vi "AlliGator Get Phasor Plot Calibration Message String.vi"(5 "Calibration CPU (s)":dbl, 6 "Calibration Phasor":T21, 7 "Message in":string, 8 "error in (no error)":errorcluster, 9 "AlliGator Phasor Calibration Options":T2={"Phasor Frequency"=0.0, "Phasor Calibration"={"Calibration Lifetime"=1e-09, "Calibration Type"=enum."Single Phasor", "Calibration Map Algorithm"=enum."Simple Search", "Use Backup Calibration if needed"=TRUE, "Backup Calibration Type"=enum."Single Calibration"}}, 10 "Phasor Calibration Map Characteristics":T1={"Phasor Frequency"=80000000.0, "Calibration Lifetime"=1e-09, "Map Resolution X"=0, "Map Resolution Y"=0, "Empty Map"=FALSE}, 11 "Phasor Plot Parameters":T5={"Phasor Frequency"=0.0, "Decay Preprocessing Options & Parameters"={"Background Subtraction Parameters"={"Background Definition Range"={"Min Gate"=0.0, "Max Gate"=0.0}, "Baseline Subtraction Method"=enum."Mean", "Background Subtraction?"=FALSE, "Background File"=path "", "Background Constant"=0.0, "Background Scaling Factor"=1.0, "Background Pile-up Correction"=FALSE, "Background Pixel Well Capacity"=1}, "Decay Preprocessing Parameters"={"Background Subtraction"=FALSE, "Straighten Decay"=FALSE, "Reverse Gates"=FALSE, "1-Normalized Decay"=FALSE, "Smoothen Decay"=FALSE, "Smoothing Parameter"=0.0, "Shift Decay"=FALSE, "Decay Shift Parameters"={"Type"=enum."Default", "Shift"=0.0, "Threshold"=0.0, "Rotate"=FALSE}, "Extrapolate Decay"=FALSE, "Additional Points"=0, "Head Fraction"=0.0, "Pixel-Normalize Decay"=FALSE, "Use Periodicity"=FALSE, "Use Cursors"=FALSE, "Tail Fraction"=0.0, "Use Decay Pre-Processing"=TRUE, "Fold Decay"=FALSE, "# Folds"=1, "[0-1]-Normalized Decay"=FALSE}, "Preprocessing Steps Order"=[]}, "FLI Dataset Modified"=FALSE, "Source Image Settings"={"Low Count Pixels Rejection Options"={"Background Low Threshold Factor"=0.0, "Fixed Low Background Threshold"=0.0, "Reject Low Count Pixels"=FALSE, "Low Percentile"=0.0}, "High Count Pixels Rejection Options"={"Background High Threshold Factor"=0.0, "Fixed High Background Threshold"=0.0, "Reject High Count Pixels"=FALSE, "High Percentile"=0.0}}, "Data Information"={"Gate Width"=0.0, "Gate Separation"=0.0, "Step (Gate Separation)"=0, "Laser Period"=0.0, "SYNC Period"=0.0, "Channel Name"=0, "Channel Arithmetic"=enum."None", "Pile-up Correction"=FALSE, "Pixel Well Capacity"=1, "Dataset Scaling Factor"=1.0}, "Phasor Plot"={"Phasor Plot Smoothing Options"={"Use Phasor Plot Smoothing"=FALSE, "Kernel Type"=enum."Uniform", "Bin"=1, "Algorithm"=enum."Rapid"}, "Phasor Plot Size"={"H"=0, "V"=0, "Margin"=0.0}, "Selected Image ROI(s)"=FALSE, "All Image ROIs"=FALSE, "Selected Source Image ROI"=0, "Source Image ROIs"=[]}} {"Phasor Plot"."Source Image ROIs"."ROI Descriptor"."Contours"."Type" items=["No Selection", "Point", "Line", "Rectangle", "Oval", "Polygon", "Freehand Region", "Annulus", "Unused2", "Unused3", "Broken Line", "Freehand Line", "Rotated Rectangle"]; "Phasor Plot"."Phasor Plot Smoothing Options"."Bin" min=1 step=2; "Data Information"."Dataset Scaling Factor" min=0.0; "Data Information"."Pixel Well Capacity" min=1 step=1; "Data Information"."Channel Name" items=["Gate"]; "Source Image Settings"."High Count Pixels Rejection Options"."High Percentile" min=0.0 max=100.0; "Source Image Settings"."Low Count Pixels Rejection Options"."Low Percentile" min=0.0 max=100.0; "Decay Preprocessing Options & Parameters"."Decay Preprocessing Parameters"."# Folds" min=1; "Decay Preprocessing Options & Parameters"."Background Subtraction Parameters"."Background Pixel Well Capacity" min=1 step=1; "Phasor Frequency" min=-2147483648.0 max=2147483647.0}) -> (0 "error out":errorcluster, 3 "Message out":string)   [LabVIEW 2021, in "AlliGator Phasor Plot.lvlib"]
doc: "Builds string specifying which phasor calibration is used."
uses:
  AlliGator Phasor Plot.lvlib
  Phasor/Calibration Phasor (m, phi).ctl
  AlliGator Phasor Plot Parameters v2.ctl
  Decay Analysis/Decay Preprocessing/AlliGator Decay Preprocessing Options.ctl
  Decay Analysis/Decay Preprocessing/AlliGator Background Subtraction Parameters.ctl
  Decay Analysis/Decay Preprocessing/AlliGator Baseline Subtraction Method.ctl
  Decay Analysis/Decay Preprocessing/AlliGator Decay Preprocessing Parameters.ctl
  Graphs/XY Graph/XY Graph Plot Shift Parameters.ctl
  Graphs/XY Graph/XY Graph Plot Shift Method.ctl
  Settings/AlliGator Low Count Pixels Rejection Options.ctl
  Settings/AlliGator High Count Pixels Rejection Options.ctl
  Settings/AlliGator Gate Arithmetic.ctl
  AlliGator Phasor Plot Smoothing Options.ctl
  Arrays/Kernel Type.ctl
  Arrays/Smoothing Algorithm.ctl
  AlliGator Phasor Plot Size.ctl
  Image/Named ROI Description.ctl
  Phasor Calibration/AlliGator Phasor Calibration Options.ctl
  Phasor/Phasor Calibration Type.ctl
  Phasor Calibration/AlliGator Calibration Map Algorithm.ctl
  Phasor/Phasor Calibration Map Characteristics.ctl
  AlliGator Abridged Phasor Plot Parameters v2.ctl
  Arrays/Arrays.lvlib
  Phasor/Phasor.lvlib
  Phasor Calibration/AlliGator Phasor Calibration.lvlib
  Variant/Variant.lvlib
  Decay Analysis/Decay Preprocessing/AlliGator Decay Preprocessing.lvlib
  Graphs/XY Graph/XY Graph Add-Ons.lvlib
  Settings/AlliGator Settings.lvlib
  Image/Image.lvlib
panel:
  # "see the AlliGator License on the block diagram (Ctrl+E or Window:Show Block Diagram)"
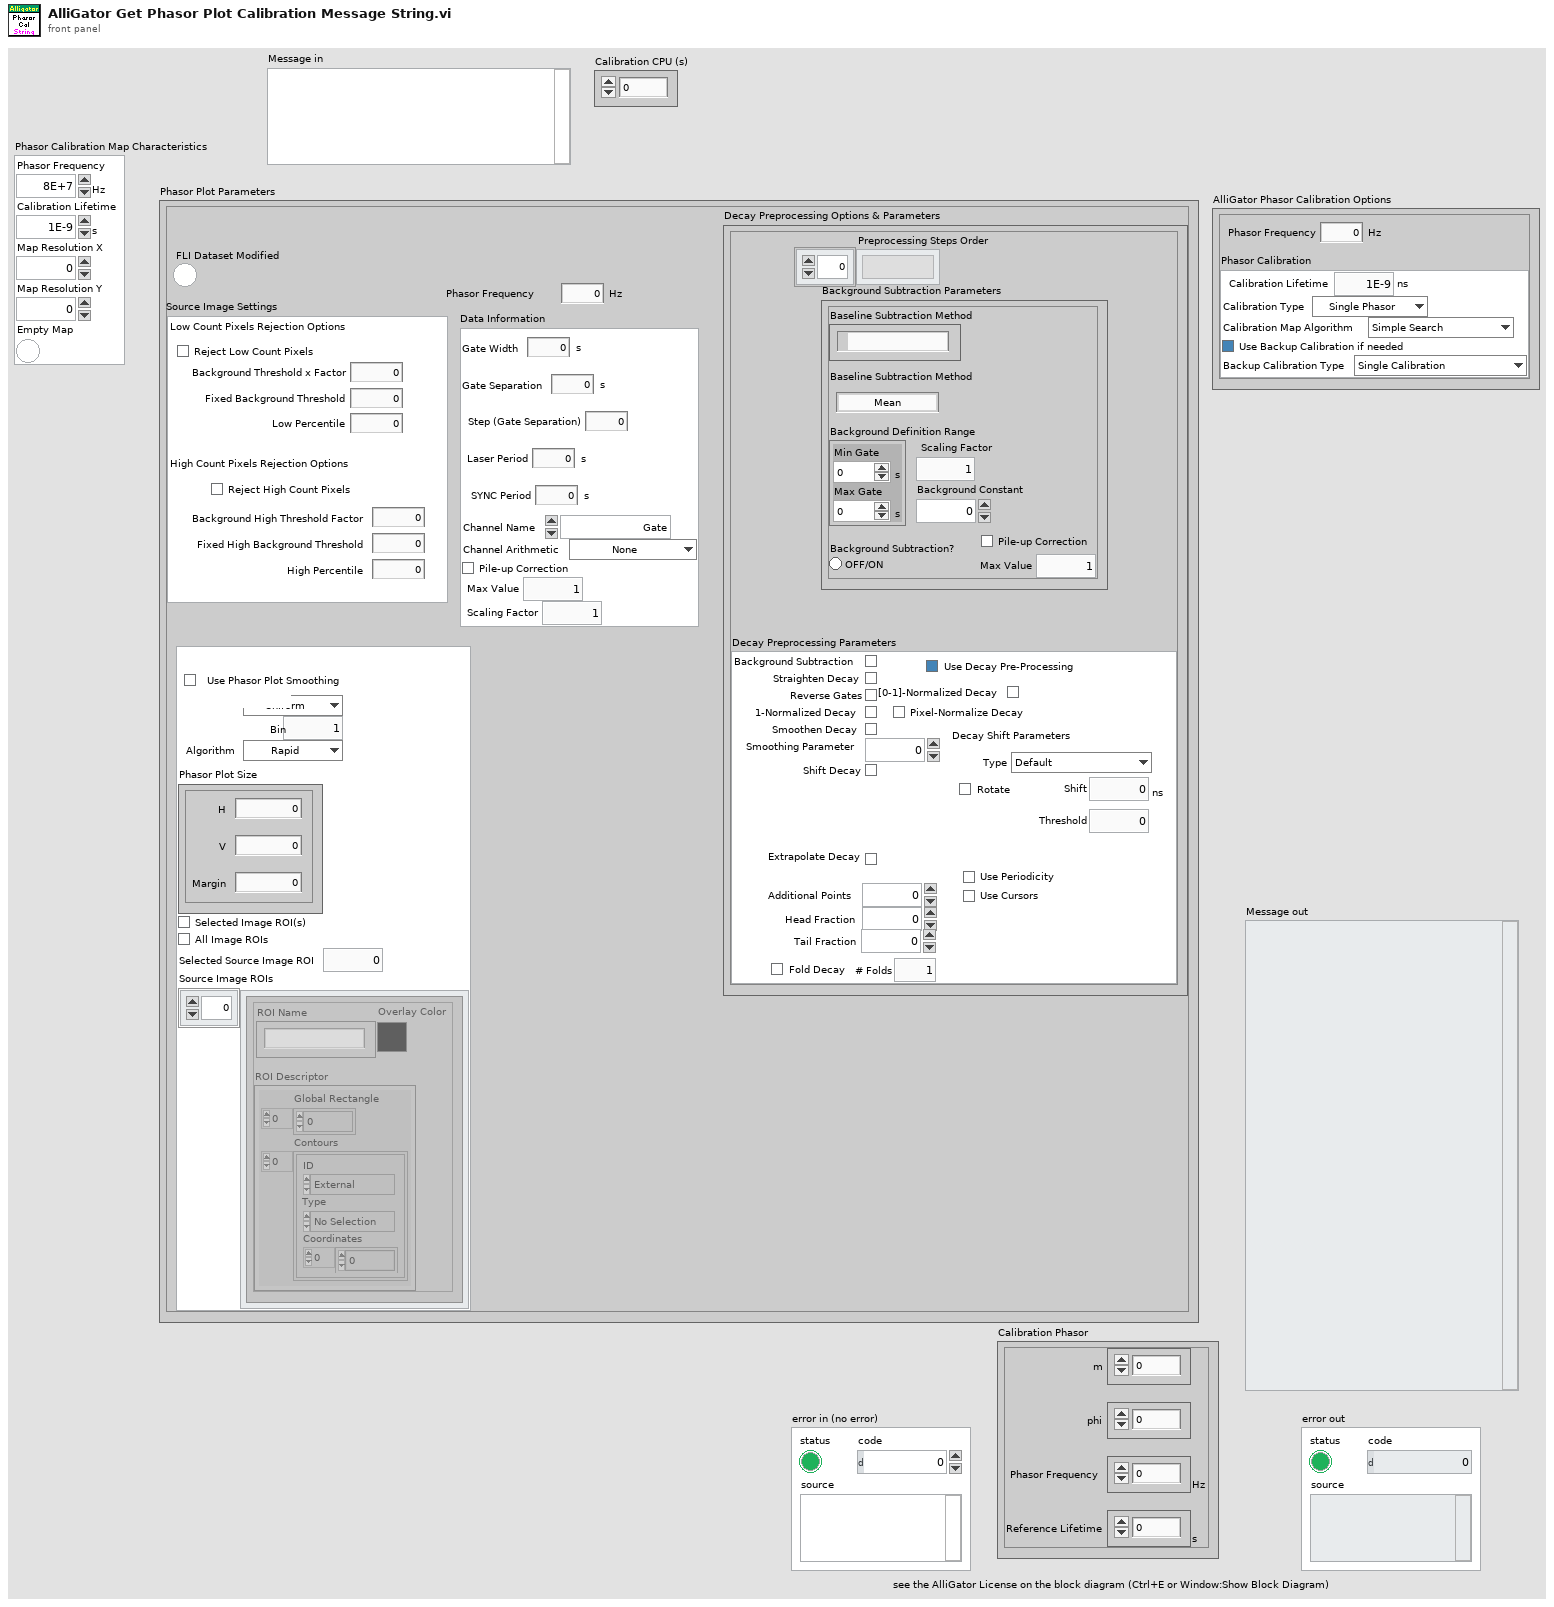
[diagram p1: front panel]
types:
  T1 = typedef "Phasor.lvlib/Phasor Calibration Map Characteristics.ctl" = cluster{"Phasor Frequency":dbl[unit], "Calibration Lifetime":dbl[unit], "Map Resolution X":i32, "Map Resolution Y":i32, "Empty Map":bool}
  T2 = typedef "AlliGator Phasor Calibration.lvlib/AlliGator Phasor Calibration Options.ctl" = cluster{"Phasor Frequency":dbl[unit], "Phasor Calibration":cluster{"Calibration Lifetime":dbl[unit], "Calibration Type":T3, "Calibration Map Algorithm":T4, "Use Backup Calibration if needed":bool, "Backup Calibration Type":enum16{"Single Calibration", "Nearest Valid Calibration"}}}
  T3 = typedef "Phasor.lvlib/Phasor Calibration Type.ctl" = enum16{"None", "Single Phasor", "Phasor Series", "Phasor Map"}
  T4 = typedef "AlliGator Phasor Calibration.lvlib/AlliGator Calibration Map Algorithm.ctl" = enum16{"Simple Search", "Min Distance"}
  T5 = typedef "AlliGator Phasor Plot.lvlib/AlliGator Phasor Plot Parameters v2.ctl" = cluster{"Phasor Frequency":dbl[unit], "Decay Preprocessing Options & Parameters":T6, "FLI Dataset Modified":bool, "Source Image Settings":cluster{"Low Count Pixels Rejection Options":T12, "High Count Pixels Rejection Options":T13}, "Data Information":cluster{"Gate Width":dbl[unit], "Gate Separation":dbl[unit], "Step (Gate Separation)":i32, "Laser Period":dbl[unit], "SYNC Period":dbl[unit], "Channel Name":u16, "Channel Arithmetic":T14, "Pile-up Correction":bool, "Pixel Well Capacity":u32, "Dataset Scaling Factor":dbl}, "Phasor Plot":cluster{"Phasor Plot Smoothing Options":T15, "Phasor Plot Size":T18, "Selected Image ROI(s)":bool, "All Image ROIs":bool, "Selected Source Image ROI":i32, "Source Image ROIs":T19[]}}
  T6 = typedef "AlliGator Decay Preprocessing.lvlib/AlliGator Decay Preprocessing Options.ctl" = cluster{"Background Subtraction Parameters":T7, "Decay Preprocessing Parameters":T9, "Preprocessing Steps Order":string[]}
  T7 = typedef "AlliGator Decay Preprocessing.lvlib/AlliGator Background Subtraction Parameters.ctl" = cluster{"Background Definition Range":cluster{"Min Gate":dbl[unit], "Max Gate":dbl[unit]}, "Baseline Subtraction Method":T8, "Background Subtraction?":bool, "Background File":path, "Background Constant":dbl, "Background Scaling Factor":dbl, "Background Pile-up Correction":bool, "Background Pixel Well Capacity":u32}
  T8 = typedef "AlliGator Decay Preprocessing.lvlib/AlliGator Baseline Subtraction Method.ctl" = enum16{"Mean", "Min", "Square Gated Single-Exponential", "File", "Constant"}
  T9 = typedef "AlliGator Decay Preprocessing.lvlib/AlliGator Decay Preprocessing Parameters.ctl" = cluster{"Background Subtraction":bool, "Straighten Decay":bool, "Reverse Gates":bool, "1-Normalized Decay":bool, "Smoothen Decay":bool, "Smoothing Parameter":dbl, "Shift Decay":bool, "Decay Shift Parameters":T10, "Extrapolate Decay":bool, "Additional Points":u32, "Head Fraction":dbl, "Pixel-Normalize Decay":bool, "Use Periodicity":bool, "Use Cursors":bool, "Tail Fraction":dbl, "Use Decay Pre-Processing":bool, "Fold Decay":bool, "# Folds":u32, "[0-1]-Normalized Decay":bool}
  T10 = typedef "XY Graph Add-Ons.lvlib/XY Graph Plot Shift Parameters.ctl" = cluster{"Type":T11, "Shift":dbl[unit], "Threshold":dbl, "Rotate":bool}
  T11 = typedef "XY Graph Add-Ons.lvlib/XY Graph Plot Shift Method.ctl" = enum16{"Default", "CFD", "Threshold", "Cross-Correlation"}
  T12 = typedef "AlliGator Settings.lvlib/AlliGator Low Count Pixels Rejection Options.ctl" = cluster{"Background Low Threshold Factor":dbl, "Fixed Low Background Threshold":dbl, "Reject Low Count Pixels":bool, "Low Percentile":dbl}
  T13 = typedef "AlliGator Settings.lvlib/AlliGator High Count Pixels Rejection Options.ctl" = cluster{"Background High Threshold Factor":dbl, "Fixed High Background Threshold":dbl, "Reject High Count Pixels":bool, "High Percentile":dbl}
  T14 = typedef "AlliGator Settings.lvlib/AlliGator Gate Arithmetic.ctl" = enum16{"None", "INT-G2", "G2/INT*<INT>", "(1 - G2/INT)*<INT>"}
  T15 = typedef "AlliGator Phasor Plot.lvlib/AlliGator Phasor Plot Smoothing Options.ctl" = cluster{"Use Phasor Plot Smoothing":bool, "Kernel Type":T16, "Bin":i32, "Algorithm":T17}
  T16 = typedef "Arrays.lvlib/Kernel Type.ctl" = enum16{"Uniform", "Bilinear", "Gaussian"}
  T17 = typedef "Arrays.lvlib/Smoothing Algorithm.ctl" = enum16{"Rapid", "Thorough"}
  T18 = typedef "AlliGator Phasor Plot.lvlib/AlliGator Phasor Plot Size.ctl" = cluster{"H":i32, "V":i32, "Margin":dbl}
  T19 = typedef "Image.lvlib/Named ROI Description.ctl" = cluster{"ROI Descriptor":T20, "ROI Name":string, "Overlay Color":u32}
  T20 = typedef "ROI Descriptor" = cluster{"Global Rectangle":i32[], "Contours":cluster{"ID":enum32{"External", "Internal"}, "Type":u32, "Coordinates":i32[]}[]}
  T21 = typedef "Phasor.lvlib/Calibration Phasor (m, phi).ctl" = cluster{"m":dbl, "phi":dbl, "Phasor Frequency":dbl[unit], "Reference Lifetime":dbl[unit]}
  T22 = typedef "AlliGator Phasor Plot.lvlib/AlliGator Abridged Phasor Plot Parameters v2.ctl" = cluster{"Phasor Frequency":dbl[unit], "Use Gate Center":bool, "Phasor Plot Smoothing Options":T15, "Selected Image ROI(s)":bool, "All Image ROIs":bool, "Calibration Lifetime":dbl[unit], "Calibration Type":T3, "Phasor Plot Size":T18, "Calibration Map Algorithm":T4, "Use Backup Calibration if needed":bool, "Backup Calibration Type":enum16{"Single Calibration", "Nearest Valid Calibration"}}
  T23 = enum16{"Single Calibration", "Nearest Valid Calibration"}
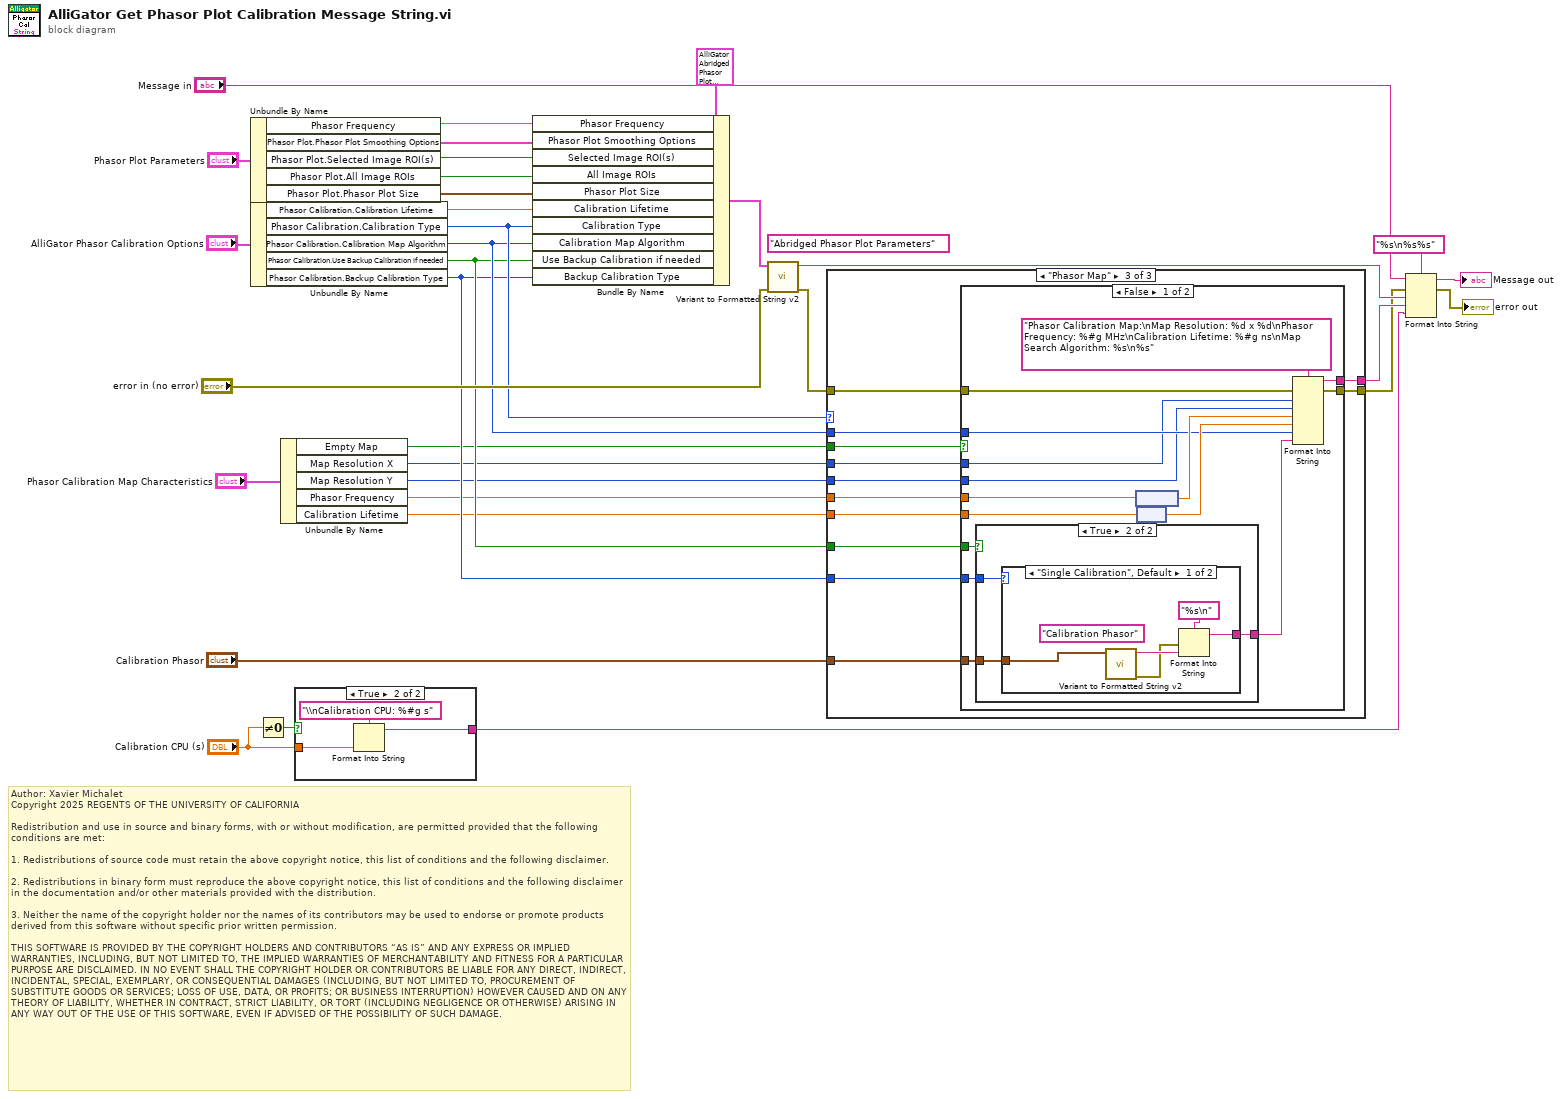
[diagram p0: block diagram]
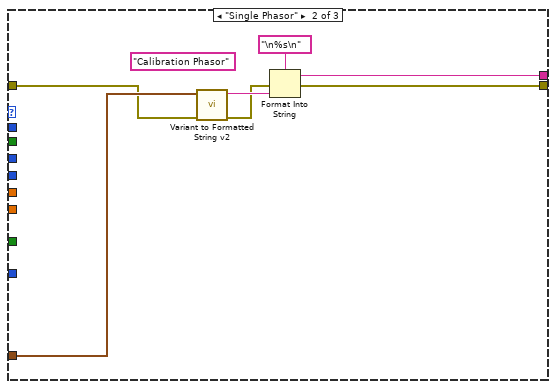
[diagram p4: hidden frame]
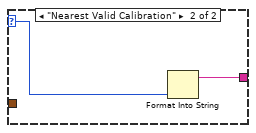
[diagram p6: hidden frame]
diagram:
  (unwired) "Abridged Phasor Plot Parameters" ("Label")
  # "Author: Xavier Michalet\nCopyright 2025 REGENTS OF THE UNIVERSITY OF CALIFORNIA\n\nRedistribution and use in source and binary forms, with or without modification, are permitted provided that the following conditions are met:\n\n1. Redistributions of source code must retain the above copyright notice, this list of conditions and the following disclaimer.\n\n2. Redistributions in binary form must reproduce the above copyright notice, this list of conditions and the following disclaimer in the documentation and/or other materials provided with the distribution.\n\n3. Neither the name of the copyright holder nor the names of its contributors may be used to endorse or promote products derived from this software without specific prior written permission.\n\nTHIS SOFTWARE IS PROVIDED BY THE COPYRIGHT HOLDERS AND CONTRIBUTORS “AS IS” AND ANY EXPRESS OR IMPLIED WARRANTIES, INCLUDING, BUT NOT LIMITED TO, THE IMPLIED WARRANTIES OF MERCHANTABILITY AND FITNESS FOR A PARTICULAR PURPOSE ARE DISCLAIMED. IN NO EVENT SHALL THE COPYRIGHT HOLDER OR CONTRIBUTORS BE LIABLE FOR ANY DIRECT, INDIRECT, INCIDENTAL, SPECIAL, EXEMPLARY, OR CONSEQUENTIAL DAMAGES (INCLUDING, BUT NOT LIMITED TO, PROCUREMENT OF SUBSTITUTE GOODS OR SERVICES; LOSS OF USE, DATA, OR PROFITS; OR BUSINESS INTERRUPTION) HOWEVER CAUSED AND ON ANY THEORY OF LIABILITY, WHETHER IN CONTRACT, STRICT LIABILITY, OR TORT (INCLUDING NEGLIGENCE OR OTHERWISE) ARISING IN ANY WAY OUT OF THE USE OF THIS SOFTWARE, EVEN IF ADVISED OF THE POSSIBILITY OF SUCH DAMAGE."
  n1 = Unbundle By Name("Phasor Plot Parameters") -> ("Phasor Frequency"=w23:dbl[unit], "Phasor Plot.Phasor Plot Smoothing Options"=w22:T15, "Phasor Plot.Selected Image ROI(s)"=w21:bool, "Phasor Plot.All Image ROIs"=w20:bool, "Phasor Plot.Phasor Plot Size"=w17:T18)
  n2 = Unbundle By Name("AlliGator Phasor Calibration Options") -> ("Phasor Calibration.Calibration Lifetime"=w15:dbl[unit], "Phasor Calibration.Calibration Type"=w14:T3, "Phasor Calibration.Calibration Map Algorithm"=w13:T4, "Phasor Calibration.Use Backup Calibration if needed"=w12:bool, "Phasor Calibration.Backup Calibration Type"=w11:T23)
  n3 = Not Equal To 0?(x="Calibration CPU (s)") -> (x != 0?=w2:bool)
  n4 = Unbundle By Name("Phasor Calibration Map Characteristics") -> ("Empty Map"=w9:bool, "Map Resolution X"=w8:i32, "Map Resolution Y"=w7:i32, "Phasor Frequency"=w6:dbl[unit], "Calibration Lifetime"=w5:dbl[unit])
  n5 = case shown="True" w2 {
    tunnel: "Calibration CPU (s)" -> [_ w36]
    tunnel: [_ w34] -> w1
    frame False {
    }
    frame True {
      n6 = Format Into String(format string="\\nCalibration CPU: %#g s", w36) -> (resulting string=w34:string)  [unwired: 2 in, 1 out]
    }
  }
  n7 = Bundle By Name(cluster=T22 {"Phasor Frequency"=0.0, "Use Gate Center"=FALSE, "Phasor Plot Smoothing Options"={"Use Phasor Plot Smoothing"=FALSE, "Kernel Type"=enum."Uniform", "Bin"=1, "Algorithm"=enum."Rapid"}, "Selected Image ROI(s)"=FALSE, "All Image ROIs"=FALSE, "Calibration Lifetime"=1e-09, "Calibration Type"=enum."Single Phasor", "Phasor Plot Size"={"H"=512, "V"=512, "Margin"=0.2}, "Calibration Map Algorithm"=enum."Simple Search", "Use Backup Calibration if needed"=TRUE, "Backup Calibration Type"=enum."Single Calibration"} ("TG Phasor Plot Parameters"), "Phasor Frequency"=w23, "Phasor Plot Smoothing Options"=w22, "Selected Image ROI(s)"=w21, "All Image ROIs"=w20, "Phasor Plot Size"=w17, "Calibration Lifetime"=w15, "Calibration Type"=w14, "Calibration Map Algorithm"=w13, "Use Backup Calibration if needed"=w12, "Backup Calibration Type"=w11) -> (w18:T22)
  n8 = call "Variant to Formatted String v2.vi"("error in (no error)"="error in (no error)", "Anything"=w18) -> ("error out"=w26:errorcluster, "String"=w32:string)  [unwired: 8 in]
  n9 = case shown="\"Phasor Map\"" w14 {
    tunnel: [_ w42 w54] -> w30
    tunnel: "Calibration Phasor" -> [_ w44 w50]
    tunnel: w26 -> [w37 w43 w56]
    tunnel: [w37 w41 w53] -> w25
    tunnel: w13 -> [_ _ w55]
    tunnel: w12 -> [_ _ w52]
    tunnel: w11 -> [_ _ w51]
    tunnel: w9 -> [_ _ w49]
    tunnel: w8 -> [_ _ w48]
    tunnel: w7 -> [_ _ w47]
    tunnel: w6 -> [_ _ w46]
    tunnel: w5 -> [_ _ w45]
    frame "None", Default {
    }
    frame "Single Phasor" {
      (unwired) "Calibration Phasor" ("Label")
      n10 = call "Variant to Formatted String v2.vi"("error in (no error)"=w43, "Anything"=w44) -> ("error out"=w39:errorcluster, "String"=w40:string)  [unwired: 8 in]
      n11 = Format Into String(format string="\n%s\n", error in=w39, w40) -> (resulting string=w42:string, error out=w41:errorcluster)  [unwired: 1 in]
    }
    frame "Phasor Map" {
      n12 = case shown="False" w49 {
        tunnel: w56 -> [w69 w82]
        tunnel: [w70 w82] -> w53
        tunnel: [w71 _] -> w54
        tunnel: w55 -> [w65 _]
        tunnel: w52 -> [w64 _]
        tunnel: w51 -> [w63 _]
        tunnel: w50 -> [w62 _]
        tunnel: w48 -> [w60 _]
        tunnel: w47 -> [w59 _]
        tunnel: w46 -> [w58 _]
        tunnel: w45 -> [w57 _]
        frame False {
          n13 = case shown="True" w64 {
            tunnel: w63 -> [_ w74]
            tunnel: w62 -> [_ w73]
            tunnel: [_ w72] -> w61
            frame False {
              # "no backup calibration used"
            }
            frame True {
              n14 = case shown="\"Single Calibration\", Default" w74 {
                selector: w74 -> [_ w81]
                tunnel: w73 -> [w76 _]
                tunnel: [w75 w80] -> w72
                frame "Single Calibration", Default {
                  (unwired) "Calibration Phasor" ("Label")
                  n15 = call "Variant to Formatted String v2.vi"("Anything"=w76) -> ("error out"=w78:errorcluster, "String"=w79:string)  [unwired: 9 in]
                  n16 = Format Into String(format string="%s\n", error in=w78, w79) -> (resulting string=w75:string)  [unwired: 1 in, 1 out]
                }
                frame "Nearest Valid Calibration" {
                  n17 = Format Into String(w81) -> (resulting string=w80:string)  [unwired: 3 in, 1 out]
                }
              }
            }
          }
          n18 = node(w58) -> (w67:dbl)
          n19 = node(w57) -> (w66:dbl)
          n20 = Format Into String(format string="Phasor Calibration Map:\nMap Resolution: %d x %d\nPhasor Frequency: %#g MHz\nCalibration Lifetime: %#g ns\nMap Search Algorithm: %s\n%s", error in=w69, w60, w59, w67, w66, w65, w61) -> (resulting string=w71:string, error out=w70:errorcluster)  [unwired: 1 in]
        }
        frame True {
          # "Empty Map"
        }
      }
    }
  }
  n21 = Format Into String(format string="%s\n%s%s", initial string="Message in", error in=w25, w32, w30, w1) -> (resulting string=→"Message out":string, error out=→"error out":errorcluster)
